vi "Save Readable Dataset.vi"   [LabVIEW 2024]
uses:
  sol-word-search/Scorer (2024Q1)/Scorer/Word Search Scorer.lvlib
types:
  T1 = enum16{"open", "replace", "create", "open or create", "replace or create", "replace or create with confirmation"}
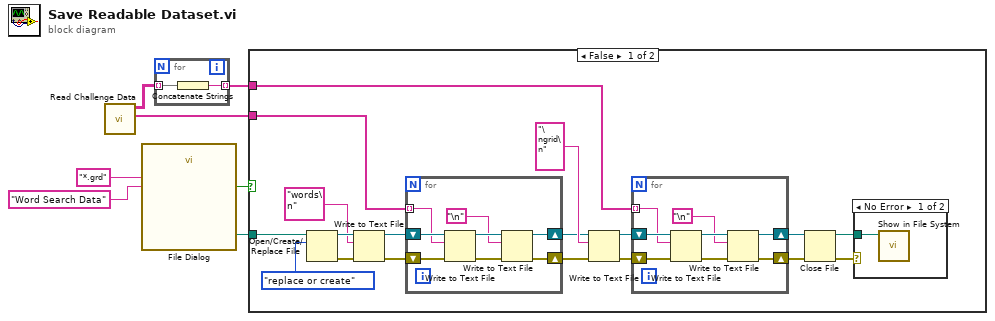
[diagram p0: block diagram]
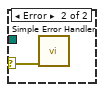
[diagram p2: hidden frame]
diagram:
  n1 = call "Read Challenge Data.vi"() -> ("Word List"=w3:string[], "Grid"=w7:string[][])  [unwired: 9 in, 1 out]
  n2 = call "File Dialog"("pattern (all files)"="*.grd", "pattern label"="Word Search Data") -> ("selected path"=w1:path, "cancelled"=w2:bool)  [unwired: 10 in, 2 out]
  n3 = for {
    tunnel: w7 -> [w9] mode=indexing
    tunnel: [w8] -> w4 mode=indexing
    n4 = Concatenate Strings(w9) -> (w8:string)
  }
  n5 = case shown="False" w2 {
    tunnel: w4 -> [w14 _]
    tunnel: w3 -> [w20 _]
    tunnel: w1 -> [w27 _]
    frame False {
      n6 = Open/Create/Replace File(file path (use dialog)=w27, operation (0:open)=T1."replace or create") -> (refnum out=w25:refnum<file>, error out=w24:errorcluster)  [unwired: 4 in, 1 out]
      n7 = Write to Text File(file (use dialog)=w25, text="words\n", error in=w24) -> (refnum out=w22:refnum<file>, error out=w21:errorcluster)  [unwired: 1 in, 1 out]
      n8 = for {
        shift-right: [w39] -> w18
        shift-left: w22 -> [w45]
        tunnel: w20 -> [w43] mode=indexing
        shift-right: [w38] -> w17
        shift-left: w21 -> [w44]
        n9 = Write to Text File(file (use dialog)=w45, text=w43, error in=w44) -> (refnum out=w42:refnum<file>, error out=w41:errorcluster)  [unwired: 1 in, 1 out]
        n10 = Write to Text File(file (use dialog)=w42, text="\n", error in=w41) -> (refnum out=w39:refnum<file>, error out=w38:errorcluster)  [unwired: 1 in, 1 out]
      }
      n11 = Write to Text File(file (use dialog)=w18, text="\ngrid\n", error in=w17) -> (refnum out=w16:refnum<file>, error out=w15:errorcluster)  [unwired: 1 in, 1 out]
      n12 = for {
        shift-right: [w31] -> w12
        shift-left: w16 -> [w37]
        tunnel: w14 -> [w35] mode=indexing
        shift-right: [w30] -> w13
        shift-left: w15 -> [w36]
        n13 = Write to Text File(file (use dialog)=w37, text=w35, error in=w36) -> (refnum out=w34:refnum<file>, error out=w33:errorcluster)  [unwired: 1 in, 1 out]
        n14 = Write to Text File(file (use dialog)=w34, text="\n", error in=w33) -> (refnum out=w31:refnum<file>, error out=w30:errorcluster)  [unwired: 1 in, 1 out]
      }
      n15 = Close File(refnum=w12, error in=w13) -> (path=w10:path, error out=w11:errorcluster)
      n16 = case shown="No Error" w11 {
        selector: w11 -> [_ w29]
        tunnel: w10 -> [w28 _]
        frame No Error {
          n17 = call <vilib>:"Show in File System.vi"("file or directory path"=w28) -> ()  [unwired: 10 in, 1 out]
        }
        frame Error {
          n18 = call <vilib>:"Simple Error Handler.vi"("error in (no error)"=w29) -> ()  [unwired: 4 in, 5 out]
        }
      }
    }
    frame True {
    }
  }
